vi "Open and Setup LIN Session.vi"(8 "error in":errorcluster, 11 "measurement configuration":T1 {"Baudrate" format="%x"; "FD Baudrate" format="%x"}) -> (0 "error out":errorcluster, 2 "session out":refnum<k21>)   [LabVIEW 2025, in "CAN-LIN Raw Bus Capture.lvclass"]
uses:
  CAN-LIN Raw Bus Capture.lvclass
  Measurement Configuration.ctl
  CAN-LIN Raw Bus Capture UI/Toggle.ctl
  <vilib>/xnet/xnet.llb/XNET Create Session (Frame Input Stream).vi
  CAN-LIN Raw Bus Capture.lvclass/CAN-LIN Raw Bus Capture.ctl
  <resource>/objmgr/xnet.rc
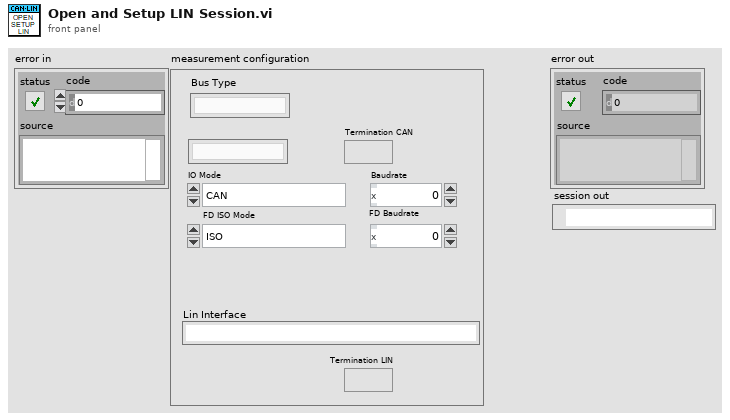
[diagram p1: front panel]
types:
  T1 = typedef "CAN-LIN Raw Bus Capture.lvclass/Measurement Configuration.ctl" = cluster{"Termination CAN":T2, "FD Baudrate":u32, "Baudrate":u32, "FD ISO Mode":enum32{"ISO", "Legacy ISO", "Non-ISO"}, "IO Mode":enum32{"CAN", "CAN FD", "CAN FD + BRS"}, "Termination LIN":T2, "Can Interface":string, "Lin Interface":string, "Bus Type":string}
  T2 = typedef "Toggle.ctl" = bool
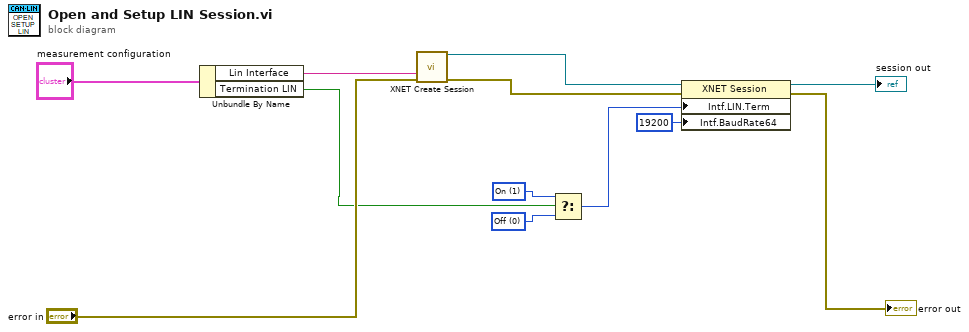
[diagram p0: block diagram]
diagram:
  w11 = u32 1 items=["Off", "On"] ("Interface:CAN:Termination")
  w12 = u32 0 items=["Off", "On"] ("Interface:CAN:Termination")
  n1 = Unbundle By Name("measurement configuration") -> ("Lin Interface"=w9:string, "Termination LIN"=w6:T2)
  n2 = call-poly <vilib>:"XNET Create Session.vi"("interface"=w9, "error in (no error)"="error in") -> ("session out"=w4:refnum<k21>, "error out"=w5:errorcluster)  [unwired: 12 in]
  n3 = Select(t=w11, s=w6, f=w12) -> (s? t:f=w10:u32)
  n4 = property class="XNET Session"(reference=w4, error in=w5, "Intf.LIN.Term"=w10, "Intf.BaudRate64"=u64 19200 ("Interface:64bit Baud Rate")) -> (reference out=→"session out":refnum<k21>, error out=→"error out":errorcluster)
